vi "Test Initialize.vi"(0 "Test Template in":refnum<class "niDTS BT Tx Test.lvclass">, 11 "error in (no error)":errorcluster) -> (4 "Test Template out":refnum<class "niDTS BT Tx Test.lvclass">, 15 "error out":errorcluster)   [LabVIEW 2015, in "niDTS BT.lvlib" / "niDTS BT Tx Test.lvclass"]
uses:
  niDTS BT Tx Test.lvclass
  RiviInstDriver/niRfsaBT/Objects/niRfsaBt.lvclass
  RiviInstDriver/niRfsaBT/Includes/niRfsaBt INC Handle.ctl
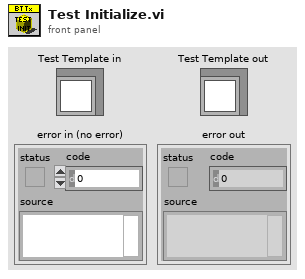
[diagram p1: front panel]
types:
  T1 = typedef "niRfsaBT.lvclass/niRfsaBT INC Handle.ctl" = refnum<data-value>
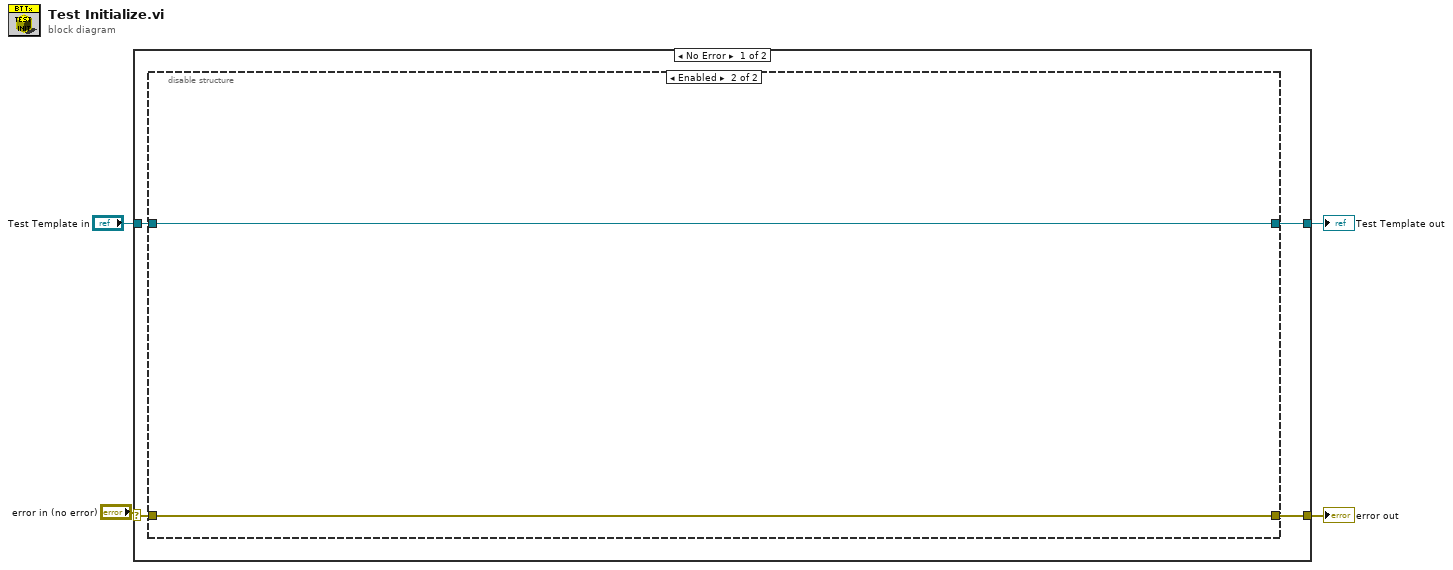
[diagram p0: block diagram]
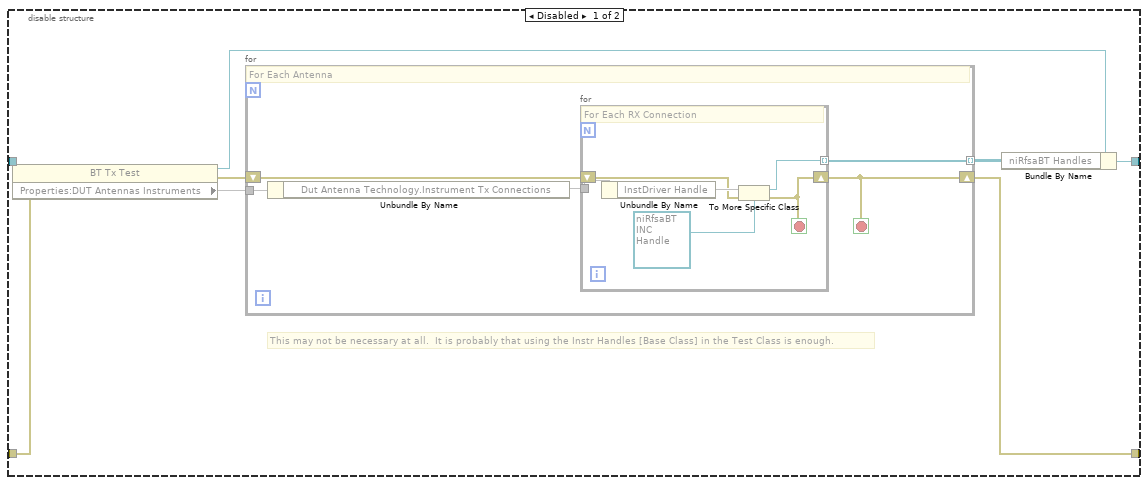
[diagram p2: hidden frame]
diagram:
  n1 = case shown="No Error" "error in (no error)" {
    selector: "error in (no error)" -> [w6 w31]
    tunnel: [w5 w31] -> w1
    tunnel: [w7 w30] -> w2
    tunnel: "Test Template in" -> [w8 w30]
    frame No Error {
      n2 = disable-structure shown="Enabled" {
        disable-tunnel: w8 -> [w13 w29]
        disable-tunnel: [w12 w29] -> w7
        disable-tunnel: w6 -> [w11 w28]
        disable-tunnel: [w10 w28] -> w5
        frame Disabled {
          # "This may not be necessary at all.  It is probably that using the Instr Handles [Base Class] in the Test Class is enough."
          n3 = property class="BT Tx Test"(reference=w13, error in=w11) -> (reference out=w14:refnum<class "niDTS BT Tx Test.lvclass">, error out=w16:errorcluster, "Properties:DUT Antennas Instruments"=w15)
          n4 = for {
            tunnel: w15 -> [w21]
            shift-right: [w18] -> w10
            shift-left: w16 -> [w19]
            tunnel: [w17] -> w9 mode=indexing
            stop <- w18 stop-if-true
            # "For Each Antenna"
            n5 = Unbundle By Name(w21) -> ("Dut Antenna Technology.Instrument Tx Connections"=w20)
            n6 = for {
              tunnel: w20 -> [w27]
              shift-right: [w24] -> w18
              shift-left: w19 -> [w25]
              tunnel: [w23] -> w17 mode=indexing
              stop <- w24 stop-if-true
              # "For Each RX Connection"
              n7 = Unbundle By Name(w27) -> ("InstDriver Handle"=w26)
              n8 = To More Specific Class(target class=T1 refnum ("niRfsaBT"), reference=w26, error in=w25) -> (specific class reference=w23:T1, error out=w24:errorcluster)
            }
          }
          n9 = Bundle By Name(cluster=w14, "niRfsaBT Handles"=w9) -> (w12:refnum<class "niDTS BT Tx Test.lvclass">)
        }
        frame Enabled {
        }
      }
    }
    frame Error {
    }
  }
  "error out" <- w1
  "Test Template out" <- w2
